vi "GenerateRandomNoise.vi"(1 "An":dbl caption="Амплитуда шума, An") -> (0 "Шум":dbl)   [LabVIEW 2019]
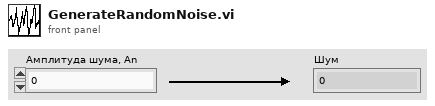
[diagram p1: front panel]
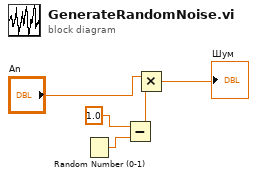
[diagram p0: block diagram]
diagram:
  n1 = Random Number (0-1)() -> (number: 0 to 1=w5:dbl)
  n2 = Subtract(x=1.0, y=w5) -> (x-y=w3:dbl)
  n3 = Multiply(x="An", y=w3) -> (x*y=→"Шум":dbl)
